vi "AIT 664 - Save Database.vi"(8 "error in (no error)":errorcluster, 11 "Node Ptr":u64 format="%.0x") -> (0 "error out":errorcluster)   [LabVIEW 2014, in "AIT 664 Custom Device.lvlib"]
doc: "Save the user defined parameters to an external file."
uses:
  AIT 664 Custom Device.lvlib
  SubVIs/Parse DB/Create Parameters Filename.vi
  SubVIs/AIT 664 - Create Database Parmeters from Sysdef Tree.vi
  SubVIs/Parse DB/AIT 664 - Parse DB.vi
  <vilib>/NI Veristand/Custom Device API/Get Item Property (Path).vi
  Controls and Global/Global.vi
  <vilib>/NI Veristand/Custom Device API/Custom Device API.lvlib
panel:
  out "empty path":bool
  out "Win File Path":string
  in  "Tag":string
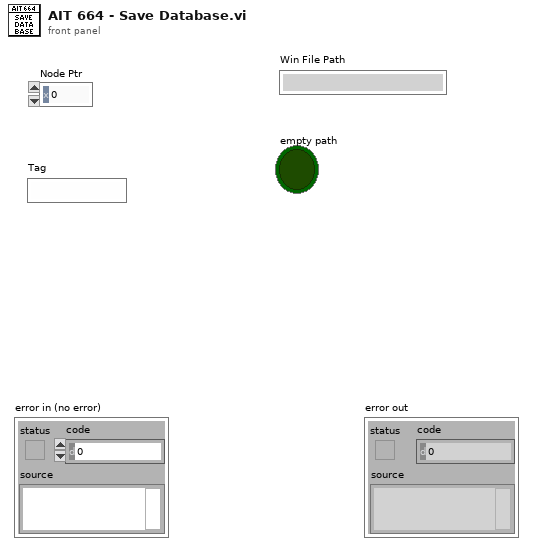
[diagram p1: front panel]
types:
  T1 = typedef "Custom Device API.lvlib/Custom Device Item Ref.ctl" = u64
  T2 = enum32{"Invalid", "Standard", "Closed", "Hidden", "Minimized", "Maximized"}
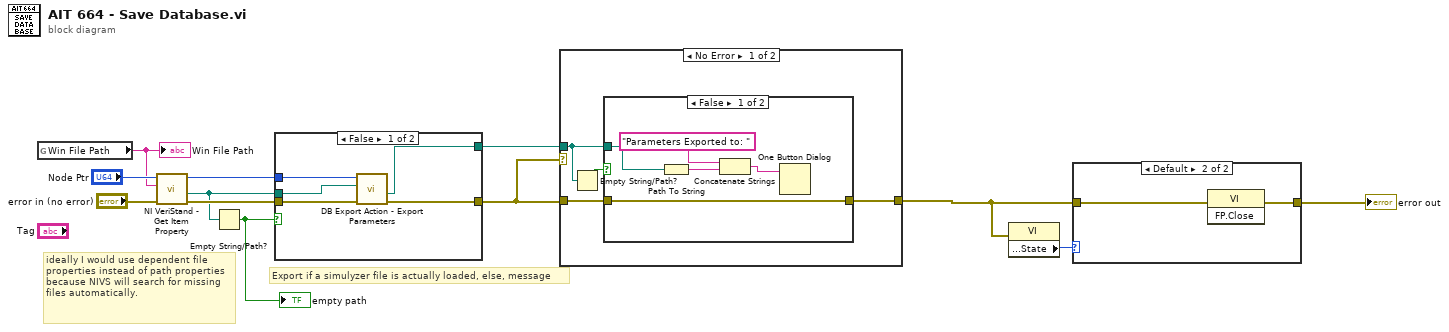
[diagram p0: block diagram]
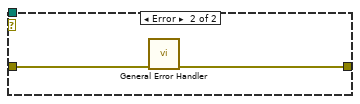
[diagram p4: hidden frame]
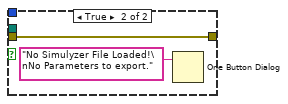
[diagram p5: hidden frame]
diagram:
  # "Export if a simulyzer file is actually loaded, else, message"
  # "ideally I would use dependent file properties instead of path properties because NIVS will search for missing files automatically."
  n1 = global read "Global.vi" "Win File Path"() -> (w8:string)
  "Win File Path" <- w8
  n2 = call-poly <vilib>:"NI VeriStand - Get Item Property.vi"("error in (no error)"="error in (no error)", "Property Name"=w8, "Item Ref in"="Node Ptr") -> ("error out"=w9:errorcluster, "Value"=w7:path, "Item Ref out"=w10:T1)  [unwired: 5 in, 1 out]
  n3 = Empty String/Path?(string/path=w7) -> (empty?=w6:bool)
  "empty path" <- w6
  n4 = case shown="False" w6 {
    tunnel: [w14 w19] -> w2
    tunnel: w9 -> [w15 w19]
    tunnel: w10 -> [w17 _]
    tunnel: w7 -> [w16 _]
    tunnel: [w13 _] -> w3
    frame False {
      n5 = call "DB Export Action - Export Parameters.vi"("error in (no error)"=w15, "selected path"=w16, "Item Ref in"=w17) -> ("error out"=w14:errorcluster, "Parm File Path"=w13:path)  [unwired: 5 in, 2 out]
    }
    frame True {
      n6 = One Button Dialog(message="No Simulyzer File Loaded!\nNo Parameters to export.") -> ()  [unwired: 1 in, 1 out]
    }
  }
  n7 = case shown="No Error" w2 {
    tunnel: w2 -> [w21 w31]
    tunnel: [w20 w30] -> w4
    tunnel: w3 -> [w22 _]
    frame No Error {
      n8 = Empty String/Path?(string/path=w22) -> (empty?=w23:bool)
      n9 = case shown="False" w23 {
        tunnel: w22 -> [w27 _]
        tunnel: w21 -> [w24 w29]
        tunnel: [w24 w29] -> w20
        frame False {
          n10 = Path To String(path=w27) -> (string=w26:string)
          n11 = Concatenate Strings("Parameters Exported to: " ("message"), w26) -> (w25:string)
          n12 = One Button Dialog(message=w25) -> ()  [unwired: 1 in, 1 out]
        }
        frame True {
        }
      }
    }
    frame Error {
      n13 = call <vilib>:"General Error Handler.vi"("error in (no error)"=w31) -> ("error out"=w30:errorcluster)  [unwired: 10 in, 4 out]
    }
  }
  n14 = property class="VI"(error in=w4) -> ("Front Panel Window:State"=w1:T2)  [unwired: 1 in, 2 out]
  n15 = case shown="Default" w1 {
    tunnel: [w32 w34] -> w5
    tunnel: w4 -> [w32 w33]
    frame "Closed" {
    }
    frame Default {
      n16 = invoke class="VI" method="FP.Close"(error in=w33) -> (error out=w34:errorcluster)  [unwired: 2 in, 2 out]
    }
  }
  "error out" <- w5
